vi "Measurement_Settings.vi"(3 "error in":errorcluster) -> (6 "out":T2, 10 "error out":errorcluster)   [LabVIEW 2010]
uses:
  X:/Software/Instruments/ISM/LabviewUnused/Utilities/controls/ctlSeqFNs_PI_SysNr.ctl
  X:/Software/Instruments/ISM/LabviewUnused/Variables/GlobalSetNumberOfDigits_PhysikalInstruments.vi
  X:/Software/Instruments/ISM/LabviewUnused/Variables/GlobalGetSetMeasurementType.vi
  X:/Software/Instruments/ISM/LabviewUnused/Variables/GlobalSetGetConfigureCamera.vi
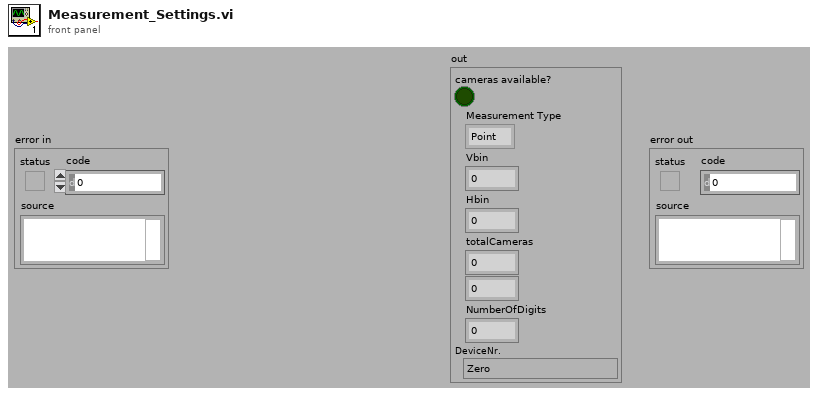
[diagram p1: front panel]
types:
  T1 = typedef "ctlSeqFNs_PI_SysNr.ctl" = enum16{"Zero", "E517", "E710"}
  T2 = cluster{"cameras available?":bool, "Measurement Type":enum16{"Point", "XDArea"}, "Vbin":i32, "Hbin":i32, "totalCameras":i32, i32, "NumberOfDigits":i32, "DeviceNr.":T1}
  T3 = cluster{bool, "Measurement Type":enum16{"Point", "XDArea"}, "Vbin":i32, "Hbin":i32, "totalCameras":i32, "totalCameras":i32, "NumberOfDigits":i32, "DeviceNr.":T1}
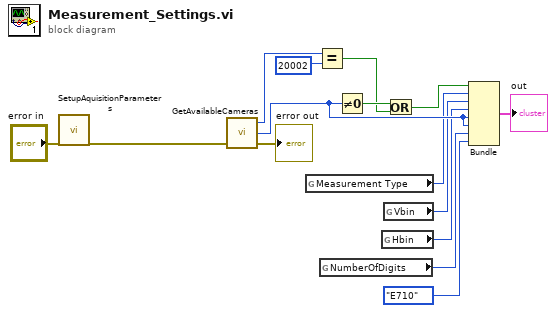
[diagram p0: block diagram]
diagram:
  n1 = call "SetupAquisitionParameters.vi"("error in"="error in") -> ("error out"=w2:errorcluster)  [unwired: 18 in]
  n2 = call "GetAvailableCameras.vi"("error in (no error)"=w2) -> ("error out"=→"error out":errorcluster, "totalCameras"=w6:i32, "DLL error code"=w12:u32)  [unwired: 2 in]
  n3 = global read "GlobalGetSetMeasurementType.vi" "Measurement Type"() -> (w5:enum16{"Point", "XDArea"})
  n4 = Equal?(x=w12, y=u32 20002) -> (x = y?=w14:bool)
  n5 = global read "GlobalSetNumberOfDigits_PhysikalInstruments.vi" "NumberOfDigits"() -> (w10:i32)
  n6 = Not Equal To 0?(x=w6) -> (x != 0?=w15:bool)
  n7 = global read "GlobalSetGetConfigureCamera.vi" "Hbin"() -> (w3:i32)
  n8 = global read "GlobalSetGetConfigureCamera.vi" "Vbin"() -> (w4:i32)
  n9 = Or(x=w15, y=w14) -> (x .or. y?=w11:bool)
  n10 = Bundle(w11, "Measurement Type"=w5, "Vbin"=w4, "Hbin"=w3, "totalCameras"=w6, "totalCameras"=w6, "NumberOfDigits"=w10, "DeviceNr."=ctlSeqFNs_PI_SysNr."E710") -> (→"out":T3)  [unwired: 1 in]
